vi "Insert.vi"(6 "Variant in":variant caption="变体输入", 7 "Shift Pressed?":bool caption="按下Shift？", 8 "error in (no error)":errorcluster caption="错误输入（无错误）", 10 "QD Combo Box Ref":refnum<vi> caption="快速放置组合框引用", 11 "QD Launch VI Ref":refnum<vi> caption="快速放置启动VI引用") -> (0 "error out":errorcluster caption="错误输出", 4 "Variant out":variant caption="变体输出")   [LabVIEW 2016]
doc: "将快速放置对话框中通过名称指定的对象放置在程序框图中所选的连线上。如同时按下[Shift]按钮，则会选中多条连线，所选对象只有一个实例被插入这些连线。\n\n默认快捷键 - [I]"
uses:
  <vilib>/Utility/miscctls.llb/LVPositionTypeDef.ctl
  <vilib>/Utility/miscctls.llb/LVPointTypeDef.ctl
panel:
  in  "Select a VI":string="选择VI..." caption="选择VI"
  in  "Undo Name":string="插入" caption="撤消名称"
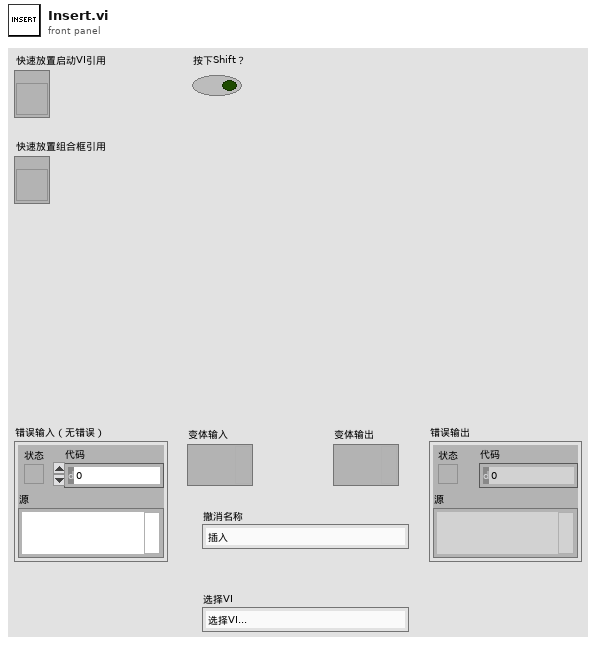
[diagram p1: front panel]
types:
  T1 = cluster{"Not Error Wire?":bool, "Source Term Top":i32, "Source Term Left":i32, "Wire Ref":refnum<vi>, "Source Term":refnum<vi>, "Sink Terms":refnum<vi>[], "Tried this one yet?":bool, "Sink Term Owner Owners":refnum<vi>[]}
  T2 = typedef "LVPositionTypeDef.ctl" = cluster{"Left":i32, "Top":i32}
  T3 = typedef "LVPointTypeDef.ctl" = cluster{"Horizontal":i16, "Vertical":i16}
  T4 = cluster{"Not Error Wire?":bool, "Source Term Top":i32, "Source Term Left":i32, "Wire Ref":refnum<vi>, "Source Term":refnum<vi>, "Sink Terms":refnum<vi>[], "Tried this one yet?":bool, "Sink Term Owner Owners":refnum<vi>[]}[]
  T5 = cluster{"Position":cluster{"h":i16, "v":i16}, "Flags":i32, "Type":enum32{"LooseEnd", "Endpoint", "Bend", "Junction"}, "Up Joint Index":i16, "Down Joint Index":i16, "Left Joint Index":i16, "Right Joint Index":i16}[]
  T6 = cluster{"Position":cluster{"h":i16, "v":i16}, "Flags":i32, "Type":enum32{"LooseEnd", "Endpoint", "Bend", "Junction"}, "Up Joint Index":i16, "Down Joint Index":i16, "Left Joint Index":i16, "Right Joint Index":i16}
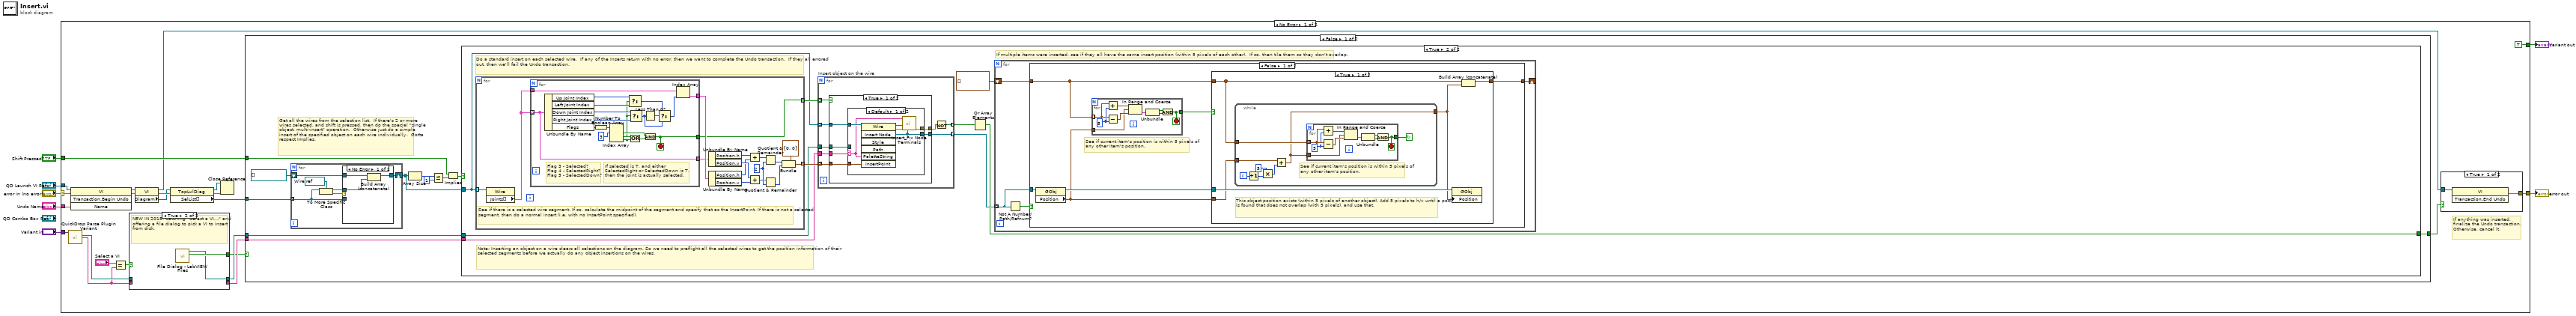
[diagram p0: block diagram]
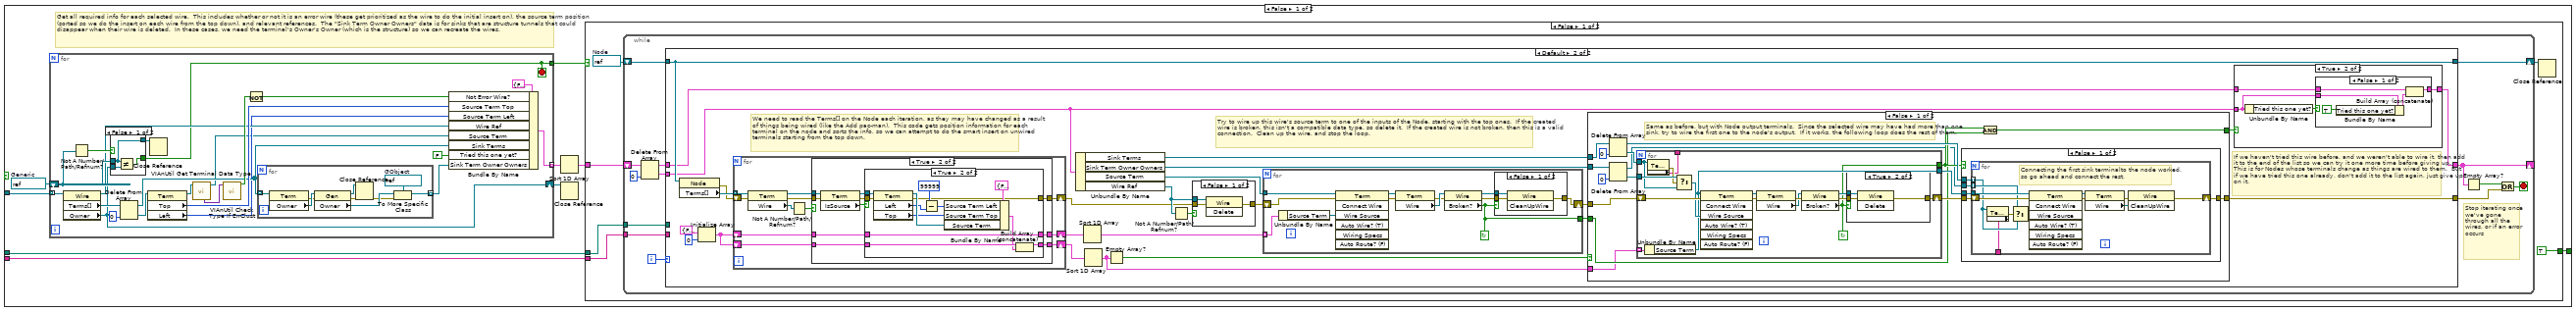
[diagram p2: hidden frame]
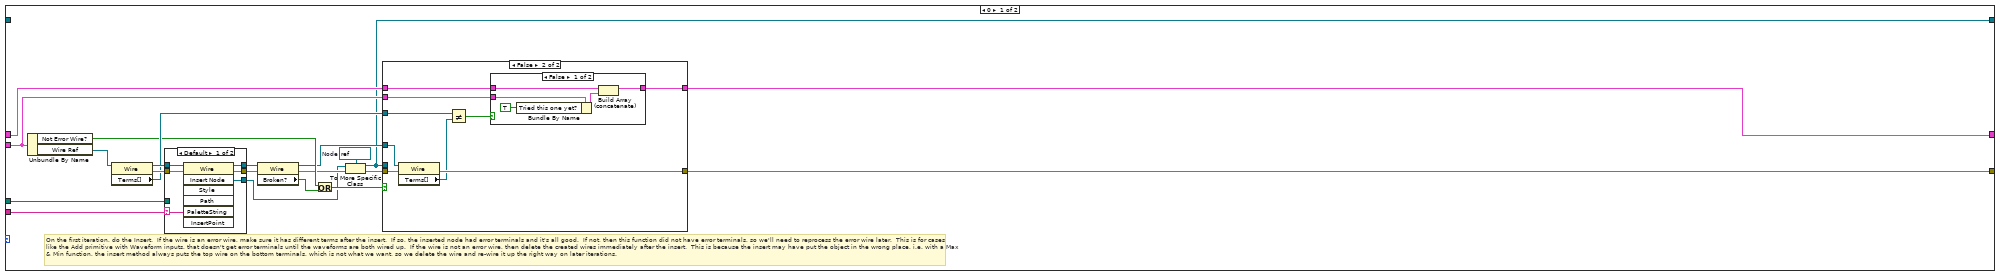
[diagram p3: hidden frame]
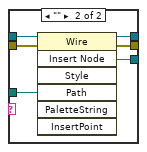
[diagram p4: hidden frame]
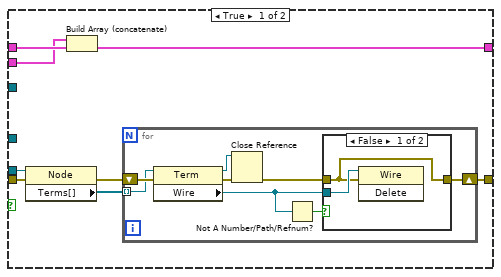
[diagram p5: hidden frame]
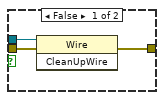
[diagram p10: hidden frame]
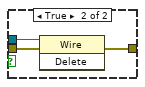
[diagram p14: hidden frame]
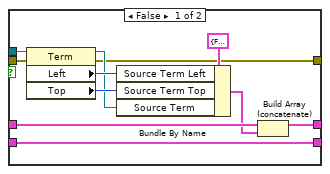
[diagram p16: hidden frame]
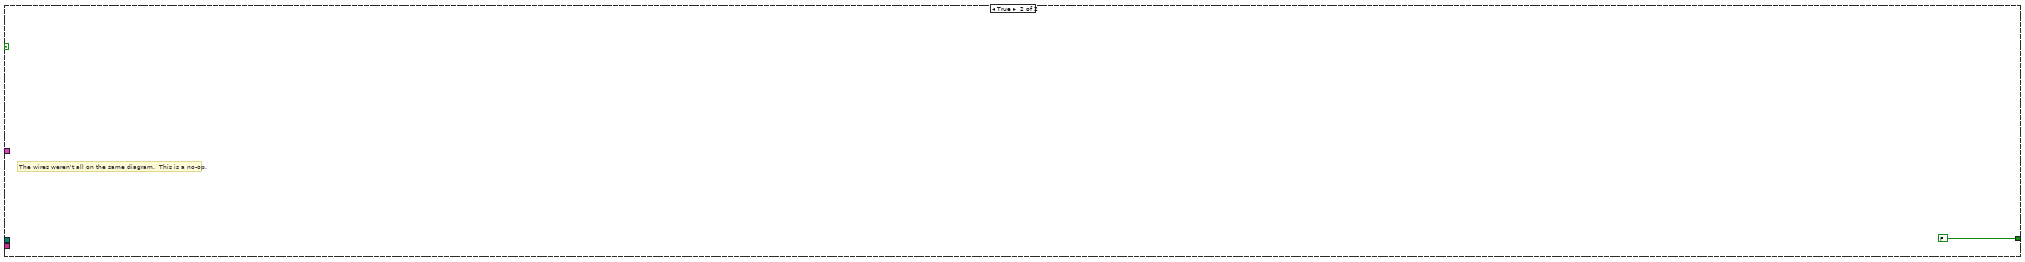
[diagram p17: hidden frame]
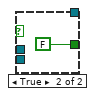
[diagram p18: hidden frame]
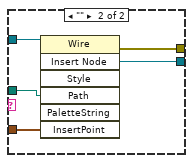
[diagram p19: hidden frame]
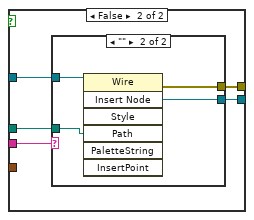
[diagram p20: hidden frame]
diagram:
  n1 = case shown="No Error" "error in (no error)" {
    selector: "error in (no error)" -> [w29 w486]
    tunnel: [w24 w486] -> w6
    tunnel: "QD Launch VI Ref" -> [w28 _]
    tunnel: "Shift Pressed?" -> [w18 _]
    tunnel: "Variant in" -> [w30 _]
    tunnel: "Undo Name" -> [w27 _]
    tunnel: [TRUE _] -> w1
    frame No Error {
      # "If anything was inserted, finalize the Undo transaction.  Otherwise, cancel it."
      n2 = call <vilib>:"QuickDrop Parse Plugin Variant.vi"("QDKS Variant in"=w30) -> ("Project VI Path"=w12:path, "Palette Object Name"=w10:string)  [unwired: 12 in, 1 out]
      n3 = invoke class="VI" method="Transaction.Begin Undo"(reference=w28, error in=w29, "Name"=w27) -> (reference out=w16:refnum<vi>, error out=w25:errorcluster)  [unwired: 1 in, 2 out]
      n4 = Equal?(x="Select a VI", y=w10) -> (x = y?=w13:bool)
      n5 = case shown="True" w13 {
        tunnel: w10 -> [w479 _]
        tunnel: w12 -> [w478 _]
        tunnel: [w479 _] -> w9
        tunnel: [w478 w480] -> w11
        tunnel: [_ w481] -> w8
        frame False {
        }
        frame True {
          # "NEW IN 2015: Catching \"Select a VI...\" and offering a file dialog to pick a VI to insert from disk."
          n6 = call <vilib>:"File Dialog - LabVIEW Files.vi"() -> ("cancelled"=w481:bool, "Path to LabVIEW File"=w480:path)  [unwired: 10 in]
        }
      }
      n7 = property class="VI"(reference=w16, error in=w25) -> (reference out=w15:refnum<vi>, error out=w23:errorcluster, "Diagram"=w22:refnum<vi>)
      n8 = property class="TopLvlDiag"(reference=w22, error in=w23) -> (reference out=w20:refnum<vi>, error out=w21:errorcluster, "SelList[]"=w19:refnum<vi>[])
      n9 = Close Reference(reference=w20, error in (no error)=w21) -> ()  [unwired: 1 out]
      n10 = case shown="False" w8 {
        tunnel: w19 -> [w41 _]
        tunnel: w18 -> [w36 _]
        tunnel: [w33 _] -> w17
        tunnel: w11 -> [w32 _]
        tunnel: w9 -> [w31 _]
        frame False {
          # "Get all the wires from the selection list.  If there's 2 or more wires selected, and shift is pressed, then do the special \"single object, multi-insert\" operation.  Otherwise just do a simple insert of the specified object on each wire individually.  Gotta respect Implies."
          n11 = for {
            tunnel: w41 -> [w469] mode=indexing
            shift-right: [w468] -> w35
            shift-left: refnum<vi>[] [] -> [w470]
            w472 = refnum<vi> refnum  # Wire
            n12 = To More Specific Class(target class=w472, reference=w469) -> (specific class reference=w467:refnum<vi>, error out=w471:errorcluster)  [unwired: 1 in]
            n13 = case shown="No Error" w471 {
              tunnel: w470 -> [w475 w477]
              tunnel: w469 -> [_ w476]
              tunnel: [w474 w477] -> w468
              tunnel: w467 -> [w473 _]
              frame No Error {
                n14 = Build Array (concatenate)(w475, w473) -> (w474:refnum<vi>[])
              }
              frame Error {
                n15 = Close Reference(reference=w476) -> ()  [unwired: 1 in, 1 out]
              }
            }
          }
          n16 = Array Size(array=w35) -> (size(s)=w39:i32)
          n17 = Less Or Equal?(x=w39, y=1) -> (x <= y?=w37:bool)
          n18 = Implies(1:w37, 2:w36) -> (0:w34:bool)
          n19 = case shown="True" w34 {
            tunnel: w31 -> [w43 w342]
            tunnel: w32 -> [w44 w341]
            tunnel: w35 -> [w46 w340]
            tunnel: [w42 w337] -> w33
            frame False {
              w49 = refnum<vi> refnum  # Generic
              # "Get all required info for each selected wire.  This includes whether or not it is an error wire (these get prioritized as the wire to do the initial insert on), the source term position (sorted so we do the insert on each wire from the top down), and relevant references.  The \"Sink Term Owner Owners\" data is for sinks that are structure tunnels that could disappear when their wire is deleted.  In these cases, we need the terminal's Owner's Owner (which is the structure) so we can recreate the wires."
              n20 = for {
                shift-right: [w308] -> w50
                shift-left: w49 -> [w323]
                tunnel: [w309] -> w48
                tunnel: w46 -> [w312] mode=indexing
                tunnel: [w311] -> w45 mode=indexing
                stop <- w309 stop-if-true
                n21 = property class="Wire"(reference=w312) -> (reference out=w315:refnum<vi>, "Terms[]"=w322:refnum<vi>[], "Owner"=w308:refnum<vi>)  [unwired: 1 in, 1 out]
                n22 = Not A Number/Path/Refnum?(number/path/refnum=w323) -> (NaN/Path/Refnum?=w320:bool)
                n23 = case shown="False" w320 {
                  tunnel: [w334 FALSE] -> w309
                  tunnel: w308 -> [w335 _]
                  tunnel: w323 -> [w333 _]
                  tunnel: [w333 _] -> w305
                  frame False {
                    n24 = Not Equal?(x=w333, y=w335) -> (x != y?=w334:bool)
                  }
                  frame True {
                  }
                }
                n25 = Delete From Array(array=w322, index=0) -> (deleted portion=w310:refnum<vi>, array with subset deleted=w307:refnum<vi>[])  [unwired: 1 in]
                n26 = property class="Term"(reference=w310) -> (reference out=w304:refnum<vi>, "Top"=w317:i32, "Left"=w306:i32)  [unwired: 1 in, 1 out]
                n27 = Close Reference(reference=w305) -> ()  [unwired: 1 in, 1 out]
                n28 = call <vilib>:"VIAnUtil Get Terminal Data Type.vi"("Terminal"=w304) -> ("dup  Terminal"=w303:refnum<vi>, "Type Variant"=w302:variant)  [unwired: 7 in, 2 out]
                n29 = call <vilib>:"VIAnUtil Check Type If ErrClust.vi"("Data In"=w302) -> ("IsErrClust?"=w318:bool)  [unwired: 1 in, 9 out]
                n30 = Not(x=w318) -> (.not. x?=w316:bool)
                n31 = for {
                  tunnel: w307 -> [w332] mode=indexing
                  tunnel: [w329] -> w313 mode=indexing
                  w328 = refnum<vi> refnum  # GObject
                  n32 = property class="Term"(reference=w332) -> (error out=w327:errorcluster, "Owner"=w331:refnum<vi>)  [unwired: 1 in, 1 out]
                  n33 = property class="Gen"(reference=w331, error in=w327) -> (reference out=w325:refnum<vi>, error out=w326:errorcluster, "Owner"=w330:refnum<vi>)
                  n34 = Close Reference(reference=w325, error in (no error)=w326) -> (error out=w324:errorcluster)
                  n35 = To More Specific Class(target class=w328, reference=w330, error in=w324) -> (specific class reference=w329:refnum<vi>)  [unwired: 1 out]
                }
                n36 = Bundle By Name(cluster=T1 {"Not Error Wire?"=FALSE, "Source Term Top"=0, "Source Term Left"=0, "Wire Ref"=refnum, "Source Term"=refnum, "Sink Terms"=[], "Tried this one yet?"=FALSE, "Sink Term Owner Owners"=[]} ("Wire Information"), "Not Error Wire?"=w316, "Source Term Top"=w317, "Source Term Left"=w306, "Wire Ref"=w315, "Source Term"=w303, "Sink Terms"=w307, "Tried this one yet?"=FALSE, "Sink Term Owner Owners"=w313) -> (w311:T1)
              }
              n37 = Sort 1D Array(array=w45) -> (sorted array=w47:T4)
              n38 = Close Reference(reference=w50) -> ()  [unwired: 1 in, 1 out]
              n39 = case shown="False" w48 {
                tunnel: w47 -> [w56 _]
                tunnel: w43 -> [w53 _]
                tunnel: w44 -> [w52 _]
                tunnel: [TRUE FALSE] -> w42
                frame False {
                  w55 = refnum<vi> refnum  # Node
                  n40 = while {
                    shift-right: [w67] -> _
                    shift-left: w56 -> [w64]
                    shift-right: [w58] -> w54
                    shift-left: w55 -> [w66]
                    tunnel: w53 -> [w60]
                    tunnel: w52 -> [w59]
                    i -> [w68]
                    stop <- w61 stop-if-true
                    # "Stop iterating once we've gone through all the wires, or if an error occurs"
                    n41 = Delete From Array(array=w64, index=0) -> (deleted portion=w69:T1, array with subset deleted=w63:T4)  [unwired: 1 in]
                    n42 = case shown="Default" w68 {
                      tunnel: w69 -> [w89 w146]
                      tunnel: w63 -> [w77 w153]
                      tunnel: [w70 w161] -> w58
                      tunnel: [w90 w152] -> w67
                      tunnel: w66 -> [_ w161]
                      tunnel: [w88 w156] -> w57
                      tunnel: w60 -> [w75 _]
                      tunnel: w59 -> [w76 _]
                      frame 0 {
                        w73 = refnum<vi> refnum  # Node
                        # "On the first iteration, do the Insert.  If the wire is an error wire, make sure it has different terms after the insert.  If so, the inserted node had error terminals and it's all good.  If not, then this function did not have error terminals, so we'll need to reprocess the error wire later.  This is for cases like the Add primitive with Waveform inputs, that doesn't get error terminals until the waveforms are both wired up.  If the wire is not an error wire, then delete the created wires immediately after the insert.  This is because the insert may have put the object in the wrong place, i.e. with a Max & Min function, the insert method always puts the top wire on the bottom terminals, which is not what we want, so we delete the wire and re-wire it up the right way on later iterations."
                        n43 = Unbundle By Name(w89) -> ("Not Error Wire?"=w83:bool, "Wire Ref"=w87:refnum<vi>)
                        n44 = property class="Wire"(reference=w87) -> (reference out=w85:refnum<vi>, error out=w86:errorcluster, "Terms[]"=w84:refnum<vi>[])  [unwired: 1 in]
                        n45 = case shown="Default" w75 {
                          selector: w75 -> [w91 _]
                          tunnel: [w96 w102] -> w71
                          tunnel: w86 -> [w95 w101]
                          tunnel: w85 -> [w94 w100]
                          tunnel: [w93 w99] -> w82
                          tunnel: [w92 w98] -> w81
                          tunnel: w76 -> [_ w97]
                          frame Default {
                            n46 = invoke class="Wire" method="Insert Node"(reference=w94, error in=w95, "PaletteString"=w91) -> (reference out=w93:refnum<vi>, error out=w92:errorcluster, "Insert Node"=w96:refnum<vi>)  [unwired: 4 in, 4 out]
                          }
                          frame "" {
                            n47 = invoke class="Wire" method="Insert Node"(reference=w100, error in=w101, "Path"=w97) -> (reference out=w99:refnum<vi>, error out=w98:errorcluster, "Insert Node"=w102:refnum<vi>)  [unwired: 4 in, 4 out]
                          }
                        }
                        n48 = property class="Wire"(reference=w82, error in=w81) -> (reference out=w80:refnum<vi>, error out=w74:errorcluster, "Broken?"=w79:bool)
                        n49 = Or(x=w83, y=w79) -> (x .or. y?=w78:bool)
                        n50 = To More Specific Class(target class=w73, reference=w71, error in=w74) -> (specific class reference=w70:refnum<vi>, error out=w72:errorcluster)
                        n51 = case shown="False" w78 {
                          tunnel: w77 -> [w110 w130]
                          tunnel: [w108 w129] -> w90
                          tunnel: w89 -> [w109 w128]
                          tunnel: [w103 w125] -> w88
                          tunnel: w72 -> [w105 w127]
                          tunnel: w80 -> [_ w126]
                          tunnel: w84 -> [_ w123]
                          tunnel: w70 -> [w106 _]
                          frame True {
                            n52 = property class="Node"(reference=w106, error in=w105) -> (error out=w107:errorcluster, "Terms[]"=w104:refnum<vi>[])  [unwired: 1 out]
                            n53 = Build Array (concatenate)(w109, w110) -> (w108:T4)
                            n54 = for {
                              shift-right: [w112] -> w103
                              shift-left: w107 -> [w118]
                              tunnel: w104 -> [w117] mode=indexing
                              n55 = property class="Term"(reference=w117, error in=w118) -> (reference out=w115:refnum<vi>, error out=w116:errorcluster, "Wire"=w111:refnum<vi>)
                              n56 = Close Reference(reference=w115, error in (no error)=w116) -> (error out=w113:errorcluster)
                              n57 = Not A Number/Path/Refnum?(number/path/refnum=w111) -> (NaN/Path/Refnum?=w114:bool)
                              n58 = case shown="False" w114 {
                                tunnel: w113 -> [w119 w121]
                                tunnel: [w119 w121] -> w112
                                tunnel: w111 -> [w120 _]
                                frame False {
                                n59 = invoke class="Wire" method="Delete"(reference=w120, error in=w119) -> ()  [unwired: 1 in, 3 out]
                                }
                                frame True {
                                }
                              }
                            }
                          }
                          frame False {
                            n60 = property class="Wire"(reference=w126, error in=w127) -> (error out=w125:errorcluster, "Terms[]"=w124:refnum<vi>[])  [unwired: 1 out]
                            n61 = Not Equal?(x=w123, y=w124) -> (x != y?=w122:bool)
                            n62 = case shown="False" w122 {
                              tunnel: w130 -> [w135 w136]
                              tunnel: [w134 w136] -> w129
                              tunnel: w128 -> [w133 _]
                              frame False {
                                n63 = Bundle By Name(cluster=w133, "Tried this one yet?"=TRUE) -> (w132:T1)
                                n64 = Build Array (concatenate)(w135, w132) -> (w134:T4)
                              }
                              frame True {
                              }
                            }
                          }
                        }
                      }
                      frame Default {
                        # "If we haven't tried this wire before, and we weren't able to wire it, then add it to the end of the list so we can try it one more time before giving up.  This is for Nodes whose terminals change as things are wired to them.  But if we have tried this one already, don't add it to the list again, just give up on it."
                        # "Try to wire up this wire's source term to one of the inputs of the Node, starting with the top ones.  If the created wire is broken, this isn't a compatible data type, so delete it.  If the created wire is not broken, then this is a valid connection.  Clean up the wire, and stop the loop."
                        # "We need to read the Terms[] on the Node each iteration, as they may have changed as a result of things being wired (like the Add pac-man).  This code gets position information for each terminal on the node and sorts the info, so we can attempt to do the smart insert on unwired terminals starting from the top down."
                        n65 = property class="Node"(reference=w161) -> (error out=w139:errorcluster, "Terms[]"=w160:refnum<vi>[])  [unwired: 1 in, 1 out]
                        n66 = Initialize Array(T1 {"Not Error Wire?"=FALSE, "Source Term Top"=0, "Source Term Left"=0, "Wire Ref"=refnum, "Source Term"=refnum, "Sink Terms"=[], "Tried this one yet?"=FALSE, "Sink Term Owner Owners"=[]} ("Wire Information"), 0) -> (w140:T4)
                        n67 = for {
                          tunnel: w160 -> [w263] mode=indexing
                          shift-right: [w259] -> w158
                          shift-left: w140 -> [w262]
                          shift-right: [w258] -> w157
                          shift-left: w140 -> [w260]
                          shift-right: [w253] -> w138
                          shift-left: w139 -> [w255]
                          n68 = property class="Term"(reference=w263, error in=w255) -> (reference out=w256:refnum<vi>, error out=w254:errorcluster, "Wire"=w257:refnum<vi>)
                          n69 = Not A Number/Path/Refnum?(number/path/refnum=w257) -> (NaN/Path/Refnum?=w261:bool)
                          n70 = case shown="True" w261 {
                            tunnel: w262 -> [w266 w274]
                            tunnel: w260 -> [w265 w273]
                            tunnel: [w266 w271] -> w259
                            tunnel: [w265 w272] -> w258
                            tunnel: w256 -> [_ w276]
                            tunnel: w254 -> [w264 w269]
                            tunnel: [w264 w267] -> w253
                            frame False {
                            }
                            frame True {
                              n71 = property class="Term"(reference=w276, error in=w269) -> (reference out=w270:refnum<vi>, error out=w268:errorcluster, "IsSource"=w275:bool)
                              n72 = case shown="True" w275 {
                                tunnel: w274 -> [w286 w298]
                                tunnel: w273 -> [w287 w300]
                                tunnel: [w287 w299] -> w272
                                tunnel: [w285 w298] -> w271
                                tunnel: w270 -> [w282 w297]
                                tunnel: w268 -> [w278 w290]
                                tunnel: [w277 w289] -> w267
                                frame False {
                                n73 = property class="Term"(reference=w282, error in=w278) -> (reference out=w279:refnum<vi>, error out=w277:errorcluster, "Left"=w281:i32, "Top"=w280:i32)
                                n74 = Bundle By Name(cluster=T1 {"Not Error Wire?"=FALSE, "Source Term Top"=0, "Source Term Left"=0, "Wire Ref"=refnum, "Source Term"=refnum, "Sink Terms"=[], "Tried this one yet?"=FALSE, "Sink Term Owner Owners"=[]} ("Wire Information"), "Source Term Left"=w281, "Source Term Top"=w280, "Source Term"=w279) -> (w283:T1)
                                n75 = Build Array (concatenate)(w286, w283) -> (w285:T4)
                                }
                                frame True {
                                n76 = property class="Term"(reference=w297, error in=w290) -> (reference out=w294:refnum<vi>, error out=w289:errorcluster, "Left"=w288:i32, "Top"=w293:i32)
                                n77 = Subtract(x=99999, y=w288) -> (x-y=w291:i32)
                                n78 = Bundle By Name(cluster=T1 {"Not Error Wire?"=FALSE, "Source Term Top"=0, "Source Term Left"=0, "Wire Ref"=refnum, "Source Term"=refnum, "Sink Terms"=[], "Tried this one yet?"=FALSE, "Sink Term Owner Owners"=[]} ("Wire Information"), "Source Term Left"=w291, "Source Term Top"=w293, "Source Term"=w294) -> (w295:T1)
                                n79 = Build Array (concatenate)(w300, w295) -> (w299:T4)
                                }
                              }
                            }
                          }
                        }
                        n80 = Unbundle By Name(w146) -> ("Sink Terms"=w145:refnum<vi>[], "Sink Term Owner Owners"=w144:refnum<vi>[], "Source Term"=w142:refnum<vi>, "Wire Ref"=w141:refnum<vi>)
                        n81 = Sort 1D Array(array=w158) -> (sorted array=w151:T4)
                        n82 = Sort 1D Array(array=w157) -> (sorted array=w150:T4)
                        n83 = Empty Array?(array=w150) -> (empty?=w143:bool)
                        n84 = Not A Number/Path/Refnum?(number/path/refnum=w141) -> (NaN/Path/Refnum?=w149:bool)
                        n85 = case shown="False" w149 {
                          tunnel: [w163 w165] -> w159
                          tunnel: w141 -> [w164 _]
                          tunnel: w138 -> [w162 w165]
                          frame False {
                            n86 = invoke class="Wire" method="Delete"(reference=w164, error in=w162) -> (error out=w163:errorcluster)  [unwired: 1 in, 2 out]
                          }
                          frame True {
                          }
                        }
                        n87 = for {
                          tunnel: w142 -> [w246]
                          tunnel: w151 -> [w245] mode=indexing
                          tunnel: [w241] -> w154
                          shift-right: [w235] -> w137
                          shift-left: w159 -> [w239]
                          stop <- w241 continue-if-true
                          n88 = Unbundle By Name(w245) -> ("Source Term"=w240:refnum<vi>)
                          n89 = invoke class="Term" method="Connect Wire"(reference=w246, error in=w239, "Wire Source"=w240) -> (reference out=w244:refnum<vi>, error out=w238:errorcluster)  [unwired: 4 in, 5 out]
                          n90 = property class="Term"(reference=w244, error in=w238) -> (error out=w237:errorcluster, "Wire"=w243:refnum<vi>)  [unwired: 1 out]
                          n91 = property class="Wire"(reference=w243, error in=w237) -> (reference out=w242:refnum<vi>, error out=w236:errorcluster, "Broken?"=w241:bool)
                          n92 = case shown="False" w241 {
                            tunnel: w242 -> [w249 w252]
                            tunnel: w236 -> [w248 w251]
                            tunnel: [w247 w250] -> w235
                            frame False {
                              n93 = invoke class="Wire" method="CleanUpWire"(reference=w249, error in=w248) -> (error out=w247:errorcluster)  [unwired: 1 in, 2 out]
                            }
                            frame True {
                              n94 = invoke class="Wire" method="Delete"(reference=w252, error in=w251) -> (error out=w250:errorcluster)  [unwired: 1 in, 2 out]
                            }
                          }
                        }
                        n95 = case shown="False" w143 {
                          tunnel: w145 -> [w181 _]
                          tunnel: [w175 w222] -> w156
                          tunnel: [w174 w223] -> w155
                          tunnel: w154 -> [w172 w223]
                          tunnel: w144 -> [w170 _]
                          tunnel: w150 -> [w167 _]
                          tunnel: w137 -> [w166 w222]
                          frame False {
                            # "Same as before, but with Node output terminals.  Since the selected wire may have had more than one sink, try to wire the first one to the node's output.  If it works, the following loop does the rest of them."
                            n96 = Delete From Array(array=w181, index=0) -> (deleted portion=w179:refnum<vi>, array with subset deleted=w176:refnum<vi>[])  [unwired: 1 in]
                            n97 = Delete From Array(array=w170, index=0) -> (deleted portion=w169:refnum<vi>, array with subset deleted=w168:refnum<vi>[])  [unwired: 1 in]
                            n98 = for {
                              tunnel: w179 -> [w201]
                              tunnel: w167 -> [w206] mode=indexing
                              shift-right: [w208] -> w178
                              shift-left: w166 -> [w215]
                              tunnel: [w203] -> w173
                              tunnel: [w204] -> w177
                              tunnel: w169 -> [w207]
                              tunnel: [w200] -> _
                              stop <- w203 continue-if-true
                              n99 = Unbundle By Name(w206) -> ("Source Term"=w204:refnum<vi>)
                              n100 = property class="Term"(reference=w201) -> (error out=w202:errorcluster, "ClassName"=w200:string)  [unwired: 1 in, 1 out]
                              n101 = Select(t=w207, s=w202, f=w201) -> (s? t:f=w205:refnum<vi>)
                              n102 = invoke class="Term" method="Connect Wire"(reference=w204, error in=w215, "Wire Source"=w205) -> (reference out=w213:refnum<vi>, error out=w214:errorcluster)  [unwired: 4 in, 5 out]
                              n103 = property class="Term"(reference=w213, error in=w214) -> (error out=w212:errorcluster, "Wire"=w211:refnum<vi>)  [unwired: 1 out]
                              n104 = property class="Wire"(reference=w211, error in=w212) -> (reference out=w209:refnum<vi>, error out=w210:errorcluster, "Broken?"=w203:bool)
                              n105 = case shown="True" w203 {
                                tunnel: w210 -> [w218 w220]
                                tunnel: w209 -> [w217 w221]
                                tunnel: [w216 w219] -> w208
                                frame False {
                                n106 = invoke class="Wire" method="CleanUpWire"(reference=w217, error in=w218) -> (error out=w216:errorcluster)  [unwired: 1 in, 2 out]
                                }
                                frame True {
                                n107 = invoke class="Wire" method="Delete"(reference=w221, error in=w220) -> (error out=w219:errorcluster)  [unwired: 1 in, 2 out]
                                }
                              }
                            }
                            n108 = case shown="False" w173 {
                              tunnel: w178 -> [w186 w199]
                              tunnel: [w183 w199] -> w175
                              tunnel: w177 -> [w185 _]
                              tunnel: w176 -> [w184 _]
                              tunnel: w168 -> [w182 _]
                              frame False {
                                n109 = for {
                                tunnel: w185 -> [w197]
                                tunnel: w184 -> [w189] mode=indexing
                                shift-right: [w187] -> w183
                                shift-left: w186 -> [w198]
                                tunnel: w182 -> [w192] mode=indexing
                                tunnel: [w188] -> _
                                # "Connecting the first sink terminalto the node worked, so go ahead and connect the rest."
                                n110 = property class="Term"(reference=w189) -> (error out=w190:errorcluster, "ClassName"=w188:string)  [unwired: 1 in, 1 out]
                                n111 = Select(t=w192, s=w190, f=w189) -> (s? t:f=w191:refnum<vi>)
                                n112 = invoke class="Term" method="Connect Wire"(reference=w197, error in=w198, "Wire Source"=w191) -> (reference out=w196:refnum<vi>, error out=w195:errorcluster)  [unwired: 4 in, 5 out]
                                n113 = property class="Term"(reference=w196, error in=w195) -> (error out=w194:errorcluster, "Wire"=w193:refnum<vi>)  [unwired: 1 out]
                                n114 = invoke class="Wire" method="CleanUpWire"(reference=w193, error in=w194) -> (error out=w187:errorcluster)  [unwired: 1 in, 2 out]
                                }
                              }
                              frame True {
                                # "None of the node outputs would connect to this wire.  No need to try to process the rest of the sinks."
                              }
                            }
                            n115 = And(x=w173, y=w172) -> (x .and. y?=w174:bool)
                          }
                          frame True {
                            # "There are no more unwired outputs on the node.  Don't bother trying to find one to wire to."
                          }
                        }
                        n116 = case shown="True" w155 {
                          tunnel: w153 -> [w224 w228]
                          tunnel: w146 -> [_ w225]
                          tunnel: [w224 w226] -> w152
                          frame False {
                          }
                          frame True {
                            n117 = Unbundle By Name(w225) -> ("Tried this one yet?"=w227:bool)
                            n118 = case shown="False" w227 {
                              tunnel: w228 -> [w233 w234]
                              tunnel: [w232 w234] -> w226
                              tunnel: w225 -> [w231 _]
                              frame False {
                                n119 = Bundle By Name(cluster=w231, "Tried this one yet?"=TRUE) -> (w230:T1)
                                n120 = Build Array (concatenate)(w233, w230) -> (w232:T4)
                              }
                              frame True {
                              }
                            }
                          }
                        }
                      }
                    }
                    n121 = Empty Array?(array=w67) -> (empty?=w62:bool)
                    n122 = Or(x=w62, y=w57) -> (x .or. y?=w61:bool)
                  }
                  n123 = Close Reference(reference=w54) -> ()  [unwired: 1 in, 1 out]
                }
                frame True {
                  # "The wires weren't all on the same diagram.  This is a no-op."
                }
              }
            }
            frame True {
              # "Note: Inserting an object on a wire clears all selections on the diagram. So we need to preflight all the selected wires to get the position information of their selected segments before we actually do any object insertions on the wires."
              # "If multiple items were inserted, see if they all have the same insert position (within 5 pixels of each other).  If so, then tile them so they don't overlap."
              # "Do a standard insert on each selected wire.  If any of the Inserts return with no error, then we want to complete the Undo transaction.  If they all errored out, then we'll fail the Undo transaction."
              n124 = for {
                tunnel: w340 -> [w447] mode=indexing
                tunnel: [w433] -> w344 mode=indexing
                tunnel: [w432] -> w343 mode=indexing
                w441 = i16 2 ("y")
                # "See if there is a selected wire segment. If so, calculate the midpoint of the segment and specify that as the InsertPoint. If there is not a selected segment, then do a normal insert (i.e. with no InsertPoint specified)."
                n125 = property class="Wire"(reference=w447) -> ("Joints[]"=w434:T5)  [unwired: 1 in, 2 out]
                n126 = for {
                  tunnel: w434 -> [w460] mode=indexing
                  tunnel: w434 -> [w459]
                  tunnel: [w460] -> w436
                  tunnel: [w458] -> w437
                  tunnel: [w448] -> w433
                  stop <- w448 stop-if-true
                  # "If selected is T, and either SelectedRight or SelectedDown is T, then the joint is actually selected."
                  # "Flag 3 - Selected?\nFlag 4 - SelectedRight?\nFlag 5 - SelectedDown?"
                  n127 = Unbundle By Name(w460) -> ("Up Joint Index"=w455:i16, "Left Joint Index"=w454:i16, "Down Joint Index"=w457:i16, "Right Joint Index"=w456:i16, "Flags"=w466:i32)
                  n128 = Number To Boolean Array(number=w466) -> (Boolean array=w465:bool[])
                  n129 = Index Array(array=w465, index #1=3 ("index")) -> (element #1=w461:bool, element #2=w462:bool, element #3=w453:bool)  [unwired: 2 in]
                  n130 = Select(t=w455, s=w453, f=w454) -> (s? t:f=w450:i16)
                  n131 = Or(x=w462, y=w453) -> (x .or. y?=w463:bool)
                  n132 = Select(t=w457, s=w453, f=w456) -> (s? t:f=w449:i16)
                  n133 = Less Than 0?(x=w449) -> (x < 0?=w451:bool)
                  n134 = And(x=w461, y=w463) -> (x .and. y?=w448:bool)
                  n135 = Select(t=w450, s=w451, f=w449) -> (s? t:f=w452:i16)
                  n136 = Index Array(array=w459, index=w452) -> (element=w458:T6)
                }
                n137 = Unbundle By Name(w436) -> ("Position.h"=w443:i16, "Position.v"=w445:i16)
                n138 = Unbundle By Name(w437) -> ("Position.h"=w444:i16, "Position.v"=w446:i16)
                n139 = Add(x=w443, y=w444) -> (x+y=w438:i16)
                n140 = Add(x=w445, y=w446) -> (x+y=w440:i16)
                n141 = Quotient & Remainder(x=w438, y=w441) -> (floor(x/y)=w439:i16)  [unwired: 1 out]
                n142 = Quotient & Remainder(x=w440, y=w441) -> (floor(x/y)=w442:i16)  [unwired: 1 out]
                n143 = Bundle(cluster=T3 {"Horizontal"=0, "Vertical"=0} ("Insertion Point"), "Horizontal"=w439, "Vertical"=w442) -> (w432:T3)
              }
              n144 = for "Insert object on the wire" {
                tunnel: w344 -> [w353] mode=indexing
                tunnel: w343 -> [w352] mode=indexing
                tunnel: w342 -> [w351]
                tunnel: w341 -> [w350]
                tunnel: w340 -> [w349] mode=indexing
                tunnel: [w348] -> w339 mode=indexing
                tunnel: [w346] -> w338 mode=indexing
                n145 = case shown="True" w353 {
                  tunnel: w351 -> [w359 w376]
                  tunnel: w350 -> [w358 w375]
                  tunnel: [w357 w374] -> w348
                  tunnel: w349 -> [w356 w373]
                  tunnel: [w355 w372] -> w347
                  tunnel: w352 -> [w354 _]
                  frame True {
                    n146 = case shown="Default" w359 {
                      selector: w359 -> [w361 _]
                      tunnel: w356 -> [w366 w371]
                      tunnel: w358 -> [_ w370]
                      tunnel: [w364 w369] -> w355
                      tunnel: [w363 w368] -> w357
                      tunnel: w354 -> [w365 w367]
                      frame Default {
                        n147 = invoke class="Wire" method="Insert Node"(reference=w366, "PaletteString"=w361, "InsertPoint"=w365) -> (reference out=w362:refnum<vi>, error out=w360:errorcluster, "Insert Node"=w363:refnum<vi>)  [unwired: 4 in, 4 out]
                        n148 = call <vilib>:"Insert_Fix Node Terminals.vi"("Inserted Node"=w363, "error in (no error)"=w360, "Original Wire"=w362, "Node Name"=w361) -> ("error out"=w364:errorcluster)  [unwired: 7 in]
                      }
                      frame "" {
                        n149 = invoke class="Wire" method="Insert Node"(reference=w371, "Path"=w370, "InsertPoint"=w367) -> (error out=w369:errorcluster, "Insert Node"=w368:refnum<vi>)  [unwired: 4 in, 5 out]
                      }
                    }
                  }
                  frame False {
                    n150 = case shown="\"\"" w376 {
                      selector: w376 -> [w377 _]
                      tunnel: w373 -> [w382 w386]
                      tunnel: w375 -> [_ w385]
                      tunnel: [w380 w384] -> w372
                      tunnel: [w379 w383] -> w374
                      frame Default {
                        n151 = invoke class="Wire" method="Insert Node"(reference=w382, "PaletteString"=w377) -> (reference out=w378:refnum<vi>, error out=w381:errorcluster, "Insert Node"=w379:refnum<vi>)  [unwired: 5 in, 4 out]
                        n152 = call <vilib>:"Insert_Fix Node Terminals.vi"("Inserted Node"=w379, "error in (no error)"=w381, "Original Wire"=w378, "Node Name"=w377) -> ("error out"=w380:errorcluster)  [unwired: 7 in]
                      }
                      frame "" {
                        n153 = invoke class="Wire" method="Insert Node"(reference=w386, "Path"=w385) -> (error out=w384:errorcluster, "Insert Node"=w383:refnum<vi>)  [unwired: 5 in, 5 out]
                      }
                    }
                  }
                }
                n154 = Not(x=w347) -> (.not. x?=w346:bool)
              }
              n155 = Or Array Elements(Boolean array=w338) -> (logical OR=w337:bool)
              n156 = for {
                tunnel: w339 -> [w388] mode=indexing
                shift-right: [w390] -> _
                shift-left: T2[] [] -> [w389]
                n157 = Not A Number/Path/Refnum?(number/path/refnum=w388) -> (NaN/Path/Refnum?=w387:bool)
                n158 = case shown="False" w387 {
                  tunnel: w388 -> [w396 _]
                  tunnel: [w395 w431] -> w390
                  tunnel: w389 -> [w393 w431]
                  frame False {
                    # "See if current item's position is within 5 pixels of any other item's position."
                    n159 = property class="GObj"(reference=w396) -> (reference out=w394:refnum<vi>, "Position"=w392:T2)  [unwired: 1 in, 1 out]
                    n160 = for {
                      tunnel: w393 -> [w405] mode=indexing
                      tunnel: w392 -> [w401]
                      tunnel: [w397] -> w391
                      stop <- w397 stop-if-true
                      w404 = 5 ("y")
                      n161 = Add(x=w405, y=w404) -> (x+y=w403:T2)
                      n162 = Subtract(x=w405, y=w404) -> (x-y=w402:T2)
                      n163 = In Range and Coerce(upper limit=w403, x=w401, lower limit=w402) -> (In Range?=w400:cluster{"Left":bool, "Top":bool})  [unwired: 1 out]
                      n164 = Unbundle(w400) -> ("Left"=w399:bool, "Top"=w398:bool)
                      n165 = And(x=w399, y=w398) -> (x .and. y?=w397:bool)
                    }
                    n166 = case shown="True" w391 {
                      tunnel: w393 -> [w409 w430]
                      tunnel: [w408 w429] -> w395
                      tunnel: w392 -> [w407 w428]
                      tunnel: w394 -> [w410 _]
                      frame True {
                        # "This object position exists (within 5 pixels of another object). Add 5 pixels to h/v until a position is found that does not overlap (with 5 pixels), and use that."
                        n167 = while {
                          tunnel: w409 -> [w413]
                          tunnel: w407 -> [w414]
                          tunnel: [w412] -> w406
                          i -> [w418]
                          stop <- w411 continue-if-true
                          # "See if current item's position is within 5 pixels of any other item's position."
                          n168 = Increment(x=w418) -> (x+1=w417:i32)
                          n169 = Multiply(x=5 ("y"), y=w417) -> (x*y=w415:i32)
                          n170 = Add(x=w414, y=w415) -> (x+y=w412:T2)
                          n171 = for {
                            tunnel: w413 -> [w427] mode=indexing
                            tunnel: w412 -> [w423]
                            tunnel: [w419] -> w411
                            stop <- w419 stop-if-true
                            w426 = 5 ("y")
                            n172 = Add(x=w427, y=w426) -> (x+y=w425:T2)
                            n173 = Subtract(x=w427, y=w426) -> (x-y=w424:T2)
                            n174 = In Range and Coerce(upper limit=w425, x=w423, lower limit=w424) -> (In Range?=w422:cluster{"Left":bool, "Top":bool})  [unwired: 1 out]
                            n175 = Unbundle(w422) -> ("Left"=w421:bool, "Top"=w420:bool)
                            n176 = And(x=w421, y=w420) -> (x .and. y?=w419:bool)
                          }
                        }
                        n177 = property class="GObj"(reference=w410, "Position"=w406) -> ()  [unwired: 1 in, 2 out]
                        n178 = Build Array (concatenate)(w409, w406) -> (w408:T2[])
                      }
                      frame False {
                        # "This object's position doesn't exist in the array. Store it to compare with later objects."
                        n179 = Build Array (concatenate)(w430, w428) -> (w429:T2[])
                      }
                    }
                  }
                  frame True {
                    # "Invalid refnum...don't bother doing anything"
                  }
                }
              }
            }
          }
        }
        frame True {
        }
      }
      n180 = case shown="True" w17 {
        tunnel: w15 -> [w482 w484]
        tunnel: [w483 w485] -> w24
        frame True {
          n181 = invoke class="VI" method="Transaction.End Undo"(reference=w482) -> (error out=w483:errorcluster)  [unwired: 2 in, 2 out]
        }
        frame False {
          n182 = invoke class="VI" method="Transaction.Fail"(reference=w484) -> (error out=w485:errorcluster)  [unwired: 2 in, 2 out]
        }
      }
    }
    frame Error {
    }
  }
  "error out" <- w6
  "Variant out" <- w1
